vi "Eye Movement Analyser.vi"(7 "Data Output":T12) -> ()   [LabVIEW 2016] (continued)
          tunnel: w2511 -> [w2526]
          tunnel: w2501 -> [w2523] mode=indexing
          shift-right: [w2525] -> w2509
          shift-left: w2507 -> [w2524]
          tunnel: w2492 -> [w2522]
          # "Delete impulses marked for deletion"
          n1237 = call "Delete Impulse.vi"("Impulse Direction +ve?"=w2527, "Number of Impulses"=w2522, "Impulse Plane"=w2526, "Impulse Positions (in)"=w2524, "Plot Number"=w2523) -> ("Impulse Positions (out)"=w2525:T11)  [unwired: 14 in]
        }
        n1238 = call "Add History.vi"("Data IN"=w2506, "Impulse Positions"=w2507) -> ("Data OUT"=w2505:T30)  [unwired: 9 in]
        n1239 = disable-structure shown="Enabled" {
          disable-tunnel: w2492 -> [w2517 w2521]
          disable-tunnel: w2501 -> [w2516 _]
          disable-tunnel: [w2514 w2521] -> w2500
          frame Disabled {
            # "Calc new No. Imp"
            # "Keep selected trace value less than number of impulses."
            n1240 = Array Size(array=w2516) -> (size(s)=w2515:i32)
            n1241 = Subtract(x=w2517, y=w2515) -> (x-y=w2514:i32)
            n1242 = local read "Trace"() -> (w2520:i32)
            n1243 = Decrement(x=w2514) -> (x-1=w2518:i32)
            n1244 = Max & Min(x=w2520, y=w2518) -> (min(x,y)=w2519:i32)  [unwired: 1 out]
            n1245 = local write "Trace"(w2519) -> ()
          }
          frame Enabled {
          }
        }
        n1246 = local write "Impulse Positions"(w2509) -> ()
        n1247 = Bundle By Name(cluster=w2505, "Impulse Positions"=w2509, "No. Imp"=w2500) -> (w2510:T30)
      }
      frame "Cut Before" {
        n1248 = local read "Impulse Plane 2"() -> (w2540:T9)
        n1249 = local read "Impulse dir"() -> (w2541:bool)
        n1250 = Unbundle By Name(w2530) -> ("Impulse Positions"=w2531:T11)
        n1251 = property on="Impulse Trace" class="WFGraph (strict)"() -> ("Cursor.Cursor Position:Cursor X"=w2537:dbl)  [unwired: 2 in, 2 out]
        n1252 = local read "Data Output"() -> (w2534:T12)
        n1253 = Unbundle By Name(w2534) -> ("Sample Rate"=w2535:i32)
        n1254 = call "Cut Impulse.vi"("Sample Rate"=w2535, "Impulse Direction +ve?"=w2541, "Cut region"=enum16{"Before", "After"}."Before", "X Position"=w2537, "Impulse Plane"=w2540, "Impulse Positions (in)"=w2531) -> ("Impulse Positions (out)"=w2538:T11)  [unwired: 13 in]
        n1255 = local write "Impulse Positions"(w2538) -> ()
        n1256 = call "Add History.vi"("Data IN"=w2530, "Impulse Positions"=w2531) -> ("Data OUT"=w2529:T30)  [unwired: 9 in]
        n1257 = Bundle By Name(cluster=w2529, "Impulse Positions"=w2538) -> (w2539:T30)
      }
      frame "Cut After" {
        n1258 = local read "Impulse Plane 2"() -> (w2555:T9)
        n1259 = local read "Data Output"() -> (w2549:T12)
        n1260 = local read "Impulse dir"() -> (w2556:bool)
        n1261 = Unbundle By Name(w2545) -> ("Impulse Positions"=w2546:T11)
        n1262 = property on="Impulse Trace" class="WFGraph (strict)"() -> ("Cursor.Cursor Position:Cursor X"=w2552:dbl)  [unwired: 2 in, 2 out]
        n1263 = Unbundle By Name(w2549) -> ("Sample Rate"=w2550:i32)
        n1264 = call "Cut Impulse.vi"("Sample Rate"=w2550, "Impulse Direction +ve?"=w2556, "Cut region"=enum16{"Before", "After"}."After", "X Position"=w2552, "Impulse Plane"=w2555, "Impulse Positions (in)"=w2546) -> ("Impulse Positions (out)"=w2553:T11)  [unwired: 13 in]
        n1265 = local write "Impulse Positions"(w2553) -> ()
        n1266 = call "Add History.vi"("Data IN"=w2545, "Impulse Positions"=w2546) -> ("Data OUT"=w2544:T30)  [unwired: 9 in]
        n1267 = Bundle By Name(cluster=w2544, "Impulse Positions"=w2553) -> (w2554:T30)
      }
      frame "Cut in Range" {
        n1268 = stacked-sequence {
          tunnel: [_ w2578 _ _] -> w2563
          tunnel: [_ _ _ w2580] -> w2564
          frame #0 {
            n1269 = property on="Time series Trace" class="WFGraph (strict)"("Active Cursor"=u32 0) -> ()  [unwired: 2 in, 2 out]
          }
          frame #1 {
            n1270 = property on="Time series Trace" class="WFGraph (strict)"() -> ("Cursor.Cursor Position:Cursor X"=w2578:dbl)  [unwired: 2 in, 2 out]
          }
          frame #2 {
            n1271 = property on="Time series Trace" class="WFGraph (strict)"("Active Cursor"=u32 1) -> ()  [unwired: 2 in, 2 out]
          }
          frame #3 {
            n1272 = property on="Time series Trace" class="WFGraph (strict)"() -> ("Cursor.Cursor Position:Cursor X"=w2580:dbl)  [unwired: 2 in, 2 out]
          }
        }
        n1273 = Unbundle By Name(w2561) -> ("Data File.Data Channels"=w2572:dbl[][], "Data File.Sample Rate"=w2567:i32)
        n1274 = Less?(x=w2563, y=w2564) -> (x < y?=w2566:bool)
        n1275 = case shown="True" w2566 {
          tunnel: w2564 -> [_ w2592]
          tunnel: w2572 -> [_ w2589]
          tunnel: [dbl[][] [] w2583] -> w2569
          tunnel: w2567 -> [_ w2582]
          frame False {
          }
          frame True {
            n1276 = Multiply(x=w2582, y=w2592) -> (x*y=w2591:dbl)
            n1277 = To Long Integer(number=w2591) -> (32bit integer=w2584:i32)
            n1278 = Array Size(array=w2589) -> (size(s)=w2588:i32[])
            n1279 = Index Array(array=w2588, index=1) -> (element=w2586:i32)
            n1280 = Subtract(x=w2586, y=w2584) -> (x-y=w2585:i32)
            n1281 = Array Subset(array=w2589, index (col)=w2584, length (col)=w2585) -> (w2590:dbl[][])  [unwired: 2 in]
            n1282 = Transpose 2D Array(2D array=w2590) -> (transposed array=w2583:dbl[][])
          }
        }
        n1283 = Multiply(x=w2567, y=w2563) -> (x*y=w2575:dbl)
        n1284 = To Long Integer(number=w2575) -> (32bit integer=w2570:i32)
        n1285 = Array Subset(array=w2572, index (col)=0 ("index"), length (col)=w2570) -> (w2574:dbl[][])  [unwired: 2 in]
        n1286 = Transpose 2D Array(2D array=w2574) -> (transposed array=w2568:dbl[][])
        n1287 = Build Array (concatenate)(w2568, w2569) -> (w2573:dbl[][])
        n1288 = Transpose 2D Array(2D array=w2573) -> (transposed array=w2565:dbl[][])
        n1289 = Bundle By Name(cluster=w2561, "Data File.Data Channels"=w2565) -> (w2560:T30)
      }
      frame "Keep in range" {
        n1290 = flat-sequence {
          tunnel: [w2611] -> w2605
          tunnel: [w2609] -> w2600
          tunnel: [w2608] -> w2599
          tunnel: w2597 -> [w2607]
          tunnel: w2605 -> [w2626]
          tunnel: [w2626] -> w2604
          tunnel: [T12 {"Data Channels"=[], "Sample Rate"=0, "Channel List"=[]} ("Data Output")] -> w2603
          tunnel: [w2624] -> w2602
          tunnel: w2599 -> [w2624]
          tunnel: [w2623] -> w2601
          tunnel: w2600 -> [w2623]
          tunnel: w2604 -> [w2628]
          tunnel: w2603 -> [w2631]
          tunnel: w2602 -> [w2630]
          tunnel: w2601 -> [w2629]
          tunnel: [w2627] -> w2595
          frame #0 {
            n1291 = Unbundle By Name(w2607) -> ("Data File.Channel List"=w2609:string[], "Data File.Data Channels"=w2613:dbl[][], "Data File.Sample Rate"=w2608:i32)
            n1292 = stacked-sequence {
              tunnel: [_ w2620 _ _] -> w2616
              tunnel: [_ _ _ w2622] -> w2615
              frame #0 {
                n1293 = property on="Time series Trace" class="WFGraph (strict)"("Active Cursor"=u32 0) -> ()  [unwired: 2 in, 2 out]
              }
              frame #1 {
                n1294 = property on="Time series Trace" class="WFGraph (strict)"() -> ("Cursor.Cursor Position:Cursor X"=w2620:dbl)  [unwired: 2 in, 2 out]
              }
              frame #2 {
                n1295 = property on="Time series Trace" class="WFGraph (strict)"("Active Cursor"=u32 1) -> ()  [unwired: 2 in, 2 out]
              }
              frame #3 {
                n1296 = property on="Time series Trace" class="WFGraph (strict)"() -> ("Cursor.Cursor Position:Cursor X"=w2622:dbl)  [unwired: 2 in, 2 out]
              }
            }
            n1297 = Subtract(x=w2615, y=w2616) -> (x-y=w2617:dbl)
            n1298 = Multiply(x=w2608, y=w2616) -> (x*y=w2612:dbl)
            n1299 = Multiply(x=w2608, y=w2617) -> (x*y=w2618:dbl)
            n1300 = To Long Integer(number=w2612) -> (32bit integer=w2614:i32)
            n1301 = To Long Integer(number=w2618) -> (32bit integer=w2610:i32)
            n1302 = Array Subset(array=w2613, index (col)=w2614, length (col)=w2610) -> (w2611:dbl[][])  [unwired: 2 in]
          }
          frame #1 {
          }
          frame #2 {
            n1303 = Bundle By Name(cluster=w2631, "Channel List"=w2629, "Data Channels"=w2628, "Sample Rate"=w2630) -> (w2627:T12)
          }
        }
        n1304 = Bundle By Name(cluster=w2597, "Data File"=w2595) -> (w2596:T30)
      }
      frame "Undo Last" {
        n1305 = Unbundle By Name(w2637) -> ("Undo Counter"=w2636:i32, "Impulse Positions"=w2638:T11)
        n1306 = case shown="0" w2636 {
          tunnel: w2638 -> [w2651 _]
          tunnel: w2637 -> [w2650 w2652]
          tunnel: [w2648 w2652] -> w2633
          frame 0 {
            n1307 = call "Add History.vi"("Data IN"=w2650, "Impulse Positions"=w2651) -> ("Data OUT"=w2649:T30)  [unwired: 9 in]
            n1308 = Bundle By Name(cluster=w2649, "Undo Counter"=1) -> (w2648:T30)
          }
          frame 1.., Default {
          }
        }
        n1309 = Unbundle By Name(w2633) -> ("Old Impulse positions for Undo"=w2644:T35, "Undo Counter"=w2635:i32, "History Length"=w2642:i32, "Histpry Position"=w2643:i32)
        n1310 = Increment(x=w2635) -> (x+1=w2639:i32)
        n1311 = Less?(x=w2639, y=w2642) -> (x < y?=w2641:bool)
        n1312 = case shown="True" w2641 {
          tunnel: w2635 -> [_ w2656]
          tunnel: w2643 -> [_ w2665]
          tunnel: w2642 -> [_ w2662]
          tunnel: w2644 -> [_ w2661]
          tunnel: w2633 -> [w2653 w2655]
          tunnel: [w2653 w2660] -> w2645
          frame False {
            n1313 = One Button Dialog(message="End of History") -> ()  [unwired: 1 in, 1 out]
          }
          frame True {
            n1314 = Subtract(x=w2665, y=w2656) -> (x-y=w2663:i32)
            n1315 = Less Than 0?(x=w2663) -> (x < 0?=w2664:bool)
            n1316 = case shown="False" w2664 {
              tunnel: w2663 -> [w2666 w2669]
              tunnel: w2662 -> [_ w2668]
              tunnel: [w2666 w2667] -> w2657
              frame False {
              }
              frame True {
                n1317 = Add(x=w2669, y=w2668) -> (x+y=w2667:i32)
              }
            }
            n1318 = Index Array(array=w2661, index (row)=w2657) -> (element=w2659:T11)  [unwired: 1 in]
            n1319 = Increment(x=w2656) -> (x+1=w2658:i32)
            n1320 = local write "Impulse Positions"(w2659) -> ()
            n1321 = Bundle By Name(cluster=w2655, "Impulse Positions"=w2659, "Undo Counter"=w2658) -> (w2660:T30)
          }
        }
      }
      frame "Redo" {
        n1322 = Unbundle By Name(w2677) -> ("Old Impulse positions for Undo"=w2676:T35, "Undo Counter"=w2672:i32, "History Length"=w2674:i32, "Histpry Position"=w2675:i32)
        n1323 = Decrement(x=w2672) -> (x-1=w2671:i32)
        n1324 = Greater Than 0?(x=w2671) -> (x > 0?=w2673:bool)
        n1325 = case shown="True" w2673 {
          tunnel: w2671 -> [_ w2686]
          tunnel: w2675 -> [_ w2694]
          tunnel: w2674 -> [_ w2691]
          tunnel: w2676 -> [_ w2690]
          tunnel: w2677 -> [w2682 w2689]
          tunnel: [w2682 w2688] -> w2680
          frame False {
            n1326 = One Button Dialog(message="Current Data") -> ()  [unwired: 1 in, 1 out]
          }
          frame True {
            n1327 = Subtract(x=w2694, y=w2686) -> (x-y=w2692:i32)
            n1328 = Less Than 0?(x=w2692) -> (x < 0?=w2693:bool)
            n1329 = case shown="True" w2693 {
              tunnel: w2692 -> [w2695 w2698]
              tunnel: w2691 -> [_ w2697]
              tunnel: [w2695 w2696] -> w2685
              frame False {
              }
              frame True {
                n1330 = Add(x=w2698, y=w2697) -> (x+y=w2696:i32)
              }
            }
            n1331 = Increment(x=w2685) -> (x+1=w2684:i32)
            n1332 = Index Array(array=w2690, index (row)=w2684) -> (element=w2687:T11)  [unwired: 1 in]
            n1333 = local write "Impulse Positions"(w2687) -> ()
            n1334 = Bundle By Name(cluster=w2689, "Impulse Positions"=w2687, "Undo Counter"=w2686) -> (w2688:T30)
          }
        }
      }
      frame "Filter Data" {
        n1335 = Unbundle By Name(w2700) -> ("Data File"=w2701:T12)
        n1336 = Unbundle By Name(w2701) -> ("Data Channels"=w2705:dbl[][], "Sample Rate"=w2711:i32)
        n1337 = local read "Interpolate"() -> (w2704:bool)
        n1338 = Unbundle By Name("Filter characteristics") -> ("Lower pass freq"=w2708:dbl, "Higher pass freq"=w2709:dbl, "Filter type"=w2712:T52, "Order"=w2710:i32)
        n1339 = case shown="True" w2704 {
          tunnel: w2705 -> [w2715 w2718]
          tunnel: [w2715 w2717] -> w2706
          frame False {
            # "Do nothing."
          }
          frame True {
            # "Interpolate without\nremoving front and end data."
            n1340 = call "interp type 2.vi"("NaN"=w2718, "Remove front and end"=FALSE) -> ("Interpolated"=w2717:dbl[][])
          }
        }
        n1341 = call "FIR filter neu.vi"("order"=w2710, "filter type"=w2712, "higher pass freq"=w2709, "lower pass freq"=w2708, "sampling freq: fs"=w2711, "3D Unfiltered Data"=w2706) -> ("Output Array"=w2707:dbl[][])  [unwired: 3 in]
        n1342 = Bundle By Name(cluster=w2700, "Data File.Data Channels"=w2707) -> (w2699:T30)
      }
      frame "Generate New Time Plot" {
        n1343 = Unbundle By Name(w2720) -> ("Data File.Sample Rate"=w2726:i32, "Parameter Time Series"=w2724:T2)
        n1344 = for {
          tunnel: w2724 -> [w2826] mode=indexing
          tunnel: w2720 -> [w2823]
          shift-right: [w2825] -> w2729
          shift-left: dbl[][] [] -> [w2824]
          tunnel: w2726 -> [w2811]
          n1345 = Unbundle By Name(w2826) -> ("List 1"=w2821:u16, "inverse"=w2820:bool, "Gain"=w2815:dbl, "Offset"=w2816:dbl, "time offset"=w2813:dbl, "interpolate"=w2808:bool)
          n1346 = Unbundle By Name(w2823) -> ("Data File.Data Channels"=w2822:dbl[][])
          n1347 = Index Array(array=w2822, index (row)=w2821) -> (element=w2817:dbl[])  [unwired: 1 in]
          n1348 = Multiply(x=w2817, y=w2815) -> (x*y=w2818:dbl[])
          n1349 = case shown="False" w2820 {
            tunnel: w2818 -> [w2830 w2832]
            tunnel: [w2830 w2831] -> w2819
            frame False {
            }
            frame True {
              n1350 = Negate(x=w2832) -> (-x=w2831:dbl[])
            }
          }
          n1351 = Add(x=w2819, y=w2816) -> (x+y=w2814:dbl[])
          n1352 = Multiply(x=w2811, y=w2813) -> (x*y=w2812:dbl)
          n1353 = Split 1D Array(array=w2814, index=w2812) -> (second subarray=w2810:dbl[])  [unwired: 1 out]
          n1354 = case shown="False" w2808 {
            tunnel: w2810 -> [w2827 w2829]
            tunnel: [w2827 w2828] -> w2809
            frame False {
            }
            frame True {
              n1355 = call "interp type 2 1D.vi"("NaN"=w2829) -> ("Interpolated"=w2828:dbl[])
            }
          }
          n1356 = Build Array (concatenate)(w2824, w2809) -> (w2825:dbl[][])
        }
        n1357 = case shown="True" "Interpolate" {
          tunnel: w2729 -> [w2732 w2735]
          tunnel: [w2732 w2734] -> w2728
          frame False {
          }
          frame True {
            n1358 = call "interp type 2.vi"("NaN"=w2735, "Remove front and end"=TRUE) -> ("Interpolated"=w2734:dbl[][])
          }
        }
        n1359 = stacked-sequence {
          tunnel: w2728 -> [_ _ w2748 _]
          tunnel: w2724 -> [_ _ _ w2792]
          tunnel: w2726 -> [_ _ w2747 _]
          tunnel: w2720 -> [_ _ w2744 _]
          frame #0 {
            n1360 = case shown="False" "Fixed Amplitude 2" {
              tunnel: [u8 0 ("Y Scale.Scale Fit") u8 2 ("Y Scale.Scale Fit")] -> w2736
              frame True {
              }
              frame False {
              }
            }
            n1361 = property on="Time series Trace" class="WFGraph (strict)"("Y Scale.Scale Fit"=w2736) -> ()  [unwired: 2 in, 2 out]
          }
          frame #1 {
            n1362 = case shown="False" "Fixed Time 2" {
              tunnel: [u8 0 ("Y Scale.Scale Fit") u8 2 ("Y Scale.Scale Fit")] -> w2741
              frame True {
              }
              frame False {
              }
            }
            n1363 = property on="Time series Trace" class="WFGraph (strict)"("X Scale.Scale Fit"=w2741) -> ()  [unwired: 2 in, 2 out]
          }
          frame #2 {
            n1364 = Reciprocal(x=w2747) -> (1/x=w2749:dbl)
            n1365 = case shown="True" "Gl Spline" {
              tunnel: w2748 -> [w2756 w2765]
              tunnel: [w2755 w2766] -> w2745
              tunnel: w2747 -> [_ w2767]
              tunnel: w2744 -> [w2754 _]
              frame False {
                n1366 = Unbundle By Name(w2754) -> ("desacc"=w2753:T31, "Data File.Sample Rate"=w2752:i32)
                n1367 = disable-structure shown="Enabled" {
                  disable-tunnel: w2756 -> [w2762 w2763]
                  disable-tunnel: [w2761 w2763] -> w2755
                  disable-tunnel: w2753 -> [w2759 _]
                  disable-tunnel: w2752 -> [w2758 _]
                  frame Disabled {
                    n1368 = call "desacade.vi"("Data not diff"=w2762, "Capture Saccades"=FALSE, "desacc"=w2759, "Sample Rate"=w2758, "Display Saccades"=FALSE) -> ("Desaccaded"=w2761:dbl[][])  [unwired: 5 in, 5 out]
                  }
                  frame Enabled {
                  }
                }
              }
              frame True {
                n1369 = local read "Interpolate"() -> (w2768:bool)
                n1370 = case shown="False" w2768 {
                  tunnel: w2765 -> [w2790 w2791]
                  tunnel: [w2789 w2791] -> w2764
                  frame False {
                    n1371 = call "interp type 2.vi"("NaN"=w2790, "Remove front and end"=TRUE) -> ("Interpolated"=w2789:dbl[][])
                  }
                  frame True {
                  }
                }
                n1372 = for {
                  tunnel: w2767 -> [w2783]
                  tunnel: w2764 -> [w2770] mode=indexing
                  tunnel: [w2772] -> w2766 mode=indexing
                  n1373 = Array Size(array=w2770) -> (size(s)=w2786:i32)
                  n1374 = Decrement(x=w2786) -> (x-1=w2785:i32)
                  n1375 = call-poly <vilib>:"Ramp Pattern.vi"("start"=0.0, "end"=w2785, "samples"=w2786) -> ("Ramp Pattern"=w2784:dbl[])  [unwired: 7 in, 1 out]
                  n1376 = Divide(x=w2784, y=w2783) -> (x/y=w2780:dbl[])
                  n1377 = call-poly <vilib>:"Mean.vi"("X"=w2770) -> ("mean"=w2771:dbl)  [unwired: 1 out]
                  n1378 = call <vilib>:"Cubic Spline Fit.vi"("Y"=w2770, "X"=w2780, "balance parameter"="Spline balance parameter") -> ("Best Cubic Spline Fit"=w2772:dbl[])  [unwired: 11 in, 1 out]
                  n1379 = Subtract(x=w2772, y=w2770) -> (x-y=w2781:dbl[])
                  n1380 = Subtract(x=w2770, y=w2771) -> (x-y=w2778:dbl[])
                  n1381 = Multiply(x=w2781, y=w2781) -> (x*y=w2782:dbl[])
                  n1382 = Multiply(x=w2778, y=w2778) -> (x*y=w2779:dbl[])
                  n1383 = Add Array Elements(numeric array=w2782) -> (sum=w2777:dbl)
                  n1384 = Add Array Elements(numeric array=w2779) -> (sum=w2776:dbl)
                  n1385 = Divide(x=w2777, y=w2776) -> (x/y=w2775:dbl)
                  n1386 = Negate(x=w2775) -> (-x=w2774:dbl)
                  n1387 = Increment(x=w2774) -> (x+1=→"R-sq":dbl)
                }
              }
            }
            n1388 = Bundle(0.0, w2749, "Best Cubic Spline Fit"=w2745) -> (→"Time series Trace":T53)  [unwired: 1 in]
          }
          frame #3 {
            n1389 = for {
              tunnel: w2792 -> [w2796] mode=indexing
              i -> [w2795]
              n1390 = Unbundle By Name(w2796) -> ("Color Box"=w2794:u32, "Boolean"=w2793:bool)
              n1391 = stacked-sequence {
                tunnel: w2795 -> [w2797 _]
                tunnel: w2793 -> [_ w2803]
                tunnel: w2794 -> [_ w2802]
                frame #0 {
                  n1392 = property on="Time series Trace" class="WFGraph (strict)"("Active Plot"=w2797) -> ()  [unwired: 2 in, 2 out]
                }
                frame #1 {
                  n1393 = local read "Interpolate"() -> (w2799:bool)
                  n1394 = case shown="False" w2799 {
                    tunnel: [u8 2 ("Plot.Point Style") u8 4 ("Plot.Point Style")] -> w2798
                    frame False {
                    }
                    frame True {
                    }
                  }
                  n1395 = case shown="False" "Dots" {
                    tunnel: [u8 0 ("Plot.Point Style") u8 2 ("Plot.Point Style")] -> w2801
                    frame False {
                    }
                    frame True {
                    }
                  }
                  n1396 = property on="Time series Trace" class="WFGraph (strict)"("Plot.Plot Color"=w2802, "Plot.Visible"=w2803, "Plot.Plot Interpolation"=w2798, "Plot.Point Style"=w2801, "Plot.Fill/Pt. Color"=w2802) -> ()  [unwired: 2 in, 2 out]
                }
              }
            }
          }
        }
        n1397 = Bundle By Name(cluster=w2723, "Session saved?"=FALSE) -> (w2722:T17)
      }
      frame "Make off and gains permanent" {
        n1398 = local read "Parameter Time Series"() -> (w2854:T2)
        n1399 = local read "Data Output"() -> (w2853:T12)
        n1400 = Unbundle By Name(w2853) -> ("Sample Rate"=w2855:i32)
        n1401 = for {
          tunnel: w2854 -> [w2873] mode=indexing
          tunnel: w2855 -> [w2863]
          shift-right: [w2857] -> w2837
          shift-left: w2853 -> [w2862]
          n1402 = Unbundle By Name(w2873) -> ("List 1"=w2860:u16, "inverse"=w2872:bool, "Gain"=w2867:dbl, "Offset"=w2868:dbl, "time offset"=w2865:dbl)
          n1403 = Unbundle By Name(w2862) -> ("Data Channels"=w2861:dbl[][])
          n1404 = Index Array(array=w2861, index (row)=w2860) -> (element=w2869:dbl[])  [unwired: 1 in]
          n1405 = Multiply(x=w2869, y=w2867) -> (x*y=w2870:dbl[])
          n1406 = case shown="True" w2872 {
            tunnel: w2870 -> [w2874 w2876]
            tunnel: [w2874 w2875] -> w2871
            frame False {
            }
            frame True {
              n1407 = Negate(x=w2876) -> (-x=w2875:dbl[])
            }
          }
          n1408 = Add(x=w2871, y=w2868) -> (x+y=w2866:dbl[])
          n1409 = Multiply(x=w2863, y=w2865) -> (x*y=w2864:dbl)
          n1410 = Split 1D Array(array=w2866, index=w2864) -> (second subarray=w2859:dbl[])  [unwired: 1 out]
          n1411 = Replace Array Subset(array=w2861, new element=w2859, index (row)=w2860) -> (w2858:dbl[][])  [unwired: 1 in]
          n1412 = Bundle By Name(cluster=w2862, "Data Channels"=w2858) -> (w2857:T12)
        }
        n1413 = File Dialog(7:"Please Enter Name Of File (NO Postfix):" ("prompt")) -> (0:w2839:errorcluster, 3:w2844:path)  [unwired: 6 in, 2 out]
        n1414 = Unbundle(w2839) -> ()  [unwired: 3 out]
        n1415 = Bundle("Data Output"=w2837, "Data OUT"=w2836) -> (w2838:T39)  [unwired: 1 in]
        n1416 = Path To String(path=w2844) -> (string=w2842:string)
        n1417 = call "File-Suffix.vi"("Substring"=".lvs-e", "String 2"=w2842) -> ("String"=w2840:string)
        n1418 = String To Path(string=w2840) -> (path=w2850:path)
        n1419 = Flatten To String(anything=w2838) -> (data string=w2847:string)  [unwired: 3 in, 2 out]
        n1420 = call <vilib>:"Open_Create_Replace File.vi"("function (open:0)"=T19."create or replace", "file path"=w2850) -> ("refnum"=w2845:refnum<file>)  [unwired: 6 in, 3 out]
        n1421 = String Length(string=w2847) -> (length=w2849:i32)
        n1422 = Flatten To String(anything=w2849) -> (data string=w2848:string)  [unwired: 3 in, 2 out]
        n1423 = call <vilib>:"Write File+ (string).vi"("string"=w2848, "refnum"=w2845) -> ("dup refnum"=w2846:refnum<file>)  [unwired: 5 in, 2 out]
        n1424 = call <vilib>:"Write File+ (string).vi"("string"=w2847, "refnum"=w2846) -> ("dup refnum"=w2852:refnum<file>)  [unwired: 5 in, 2 out]
        n1425 = call <vilib>:"Close File+.vi"("refnum"=w2852) -> ()  [unwired: 4 in, 3 out]
      }
      frame "Export Data" {
        n1426 = stacked-sequence {
          seq-local: [w2899 _] -> [_ w2966]
          seq-local: [w2895 _] -> [_ w2959]
          tunnel: w2880 -> [w2905 _]
          frame #0 {
            w2893 = TRUE ("Mean and STD")
            (unwired) T54."new or existing file" ("select mode (2)")
            w2906 = "\r"
            w2922 = "\r"
            n1427 = local read "Parameter Impuls Series"() -> (w2930:T8)
            n1428 = local read "Data Output"() -> (w2884:T12)
            n1429 = Unbundle By Name(w2905) -> ("Impulse Positions"=w2933:T11, "desacc"=w2882:T31)
            n1430 = Unbundle By Name(w2884) -> ("Sample Rate"=w2885:i32, "Channel List"=w2883:string[])
            n1431 = Index Array(array=w2930, index=0 ("Index")) -> (element=w2928:T55)
            n1432 = Array Size(array=w2883) -> (size(s)=w2918:i32)
            n1433 = for {
              tunnel: w2928 -> [w2946]
              tunnel: [w2945] -> w2927 mode=indexing
              shift-right: [w2943] -> w2907
              shift-left: "" -> [w2944]
              tunnel: w2883 -> [w2942] mode=indexing
              i -> [w2938]
              n1434 = local read "Parameter Impuls Series"() -> (w2939:T8)
              n1435 = for {
                tunnel: w2939 -> [w2953] mode=indexing
                tunnel: w2938 -> [w2951]
                shift-right: [w2948] -> w2936
                shift-left: FALSE ("Boolean 3") -> [w2949]
                n1436 = Unbundle By Name(w2953) -> ("Channel"=w2952:u16, "Desaccade"=w2947:bool)
                n1437 = Equal?(x=w2951, y=w2952) -> (x = y?=w2950:bool)
                n1438 = case shown="True" w2950 {
                  tunnel: w2949 -> [w2954 _]
                  tunnel: [w2954 w2955] -> w2948
                  tunnel: w2947 -> [_ w2955]
                  frame False {
                  }
                  frame True {
                  }
                }
              }
              n1439 = Bundle By Name(cluster=w2946, "Gain"=1.0, "Offset"=0.0, "Invert"=FALSE ("Boolean 2"), "Channel"=w2938, "Desaccade"=w2936) -> (w2945:T55)
              n1440 = Concatenate Strings(w2944, w2942, "\t") -> (w2943:string)
            }
            n1441 = Format Into String(format string="%d" ("Format String"), w2918) -> (resulting string=w2916:string)  [unwired: 2 in, 1 out]
            n1442 = local read "Impulse Plane 2"() -> (w2931:T9)
            n1443 = local read "Impulse dir"() -> (w2932:bool)
            n1444 = To Double Precision Float(number=w2885) -> (double precision float=w2926:dbl)
            n1445 = local read "Interpolate"() -> (w2889:bool)
            n1446 = Unbundle By Name(w2884) -> ("Sample Rate"=w2896:i32, "Channel List"=w2897:string[])
            n1447 = Format Into String(format string="%d" ("Format String"), w2926) -> (resulting string=w2924:string)  [unwired: 2 in, 1 out]
            n1448 = local read "S-pline"() -> (w2886:bool)
            n1449 = Concatenate Strings("Number of Channels " ("Substring"), w2916, w2906, "Channel  Names " ("Substring"), w2906, w2907) -> (w2923:string)
            n1450 = Concatenate Strings("Sample Rate ", w2924, w2922, w2923, w2922) -> (w2909:string)
            n1451 = local read "Spline balance parameter"() -> (w2887:dbl)
            n1452 = call "Couple Head Impulse Traces.vi"("Data Input"=w2884, "Impulse Positions"=w2933, "Impulse Direction +ve?"=w2932, "Impulse Plane"=w2931, "Mean and STD"=w2893, "Plot Selection 2"=w2927, "Export"=w2893, "desacc"=w2882, "Interpolate"=w2889, "S-pline"=w2886, "balance parameter (s-pline Parameter)"=w2887) -> ("Mean and STD"=w2894:dbl[][])  [unwired: 5 in, 3 out]
            n1453 = File Dialog(7:"Please Enter Name Of File (NO Postfix):" ("prompt")) -> (0:w2888:errorcluster, 3:w2899:path)  [unwired: 6 in, 2 out]
            n1454 = Transpose 2D Array "Means"(2D array=w2894) -> (transposed array=w2915:dbl[][])
            n1455 = local read "Data Output"() -> (w2898:T12)
            n1456 = Bundle By Name(cluster=w2898, "Data Channels"=w2894, "Sample Rate"=w2896, "Channel List"=w2897) -> (w2895:T12)
            n1457 = Unbundle(w2888) -> ()  [unwired: 3 out]
            n1458 = Path To String(path=w2899) -> (string=w2891:string)
            n1459 = call "File-Suffix.vi"("Substring"=".txt", "String 2"=w2891) -> ("String"=w2890:string)
            n1460 = Array To Spreadsheet String(delimiter (Tab)="\t", array=w2915, 3:"%.5f" ("format string")) -> (spreadsheet string=w2912:string)
            n1461 = String To Path(string=w2890) -> (path=w2900:path)
            n1462 = call <vilib>:"Open_Create_Replace File.vi"("function (open:0)"=T19."create or replace", "file path"=w2900) -> ("error out"=w2904:errorcluster, "refnum"=w2903:refnum<file>)  [unwired: 6 in, 2 out]
            n1463 = call <vilib>:"Write File+ (string).vi"("string"=w2909, "error in (no error)"=w2904, "refnum"=w2903) -> ("dup refnum"=w2911:refnum<file>)  [unwired: 4 in, 2 out]
            n1464 = call <vilib>:"Write File+ (string).vi"("string"=w2912, "refnum"=w2911) -> ("dup refnum"=w2910:refnum<file>)  [unwired: 5 in, 2 out]
            n1465 = call <vilib>:"Close File+.vi"("refnum"=w2910) -> ()  [unwired: 4 in, 3 out]
          }
          frame #1 {
            n1466 = Path To String(path=w2966) -> (string=w2957:string)
            n1467 = call "File-Suffix.vi"("Substring"=".lvd", "String 2"=w2957) -> ("String"=w2958:string)
            n1468 = String To Path(string=w2958) -> (path=w2965:path)
            n1469 = Flatten To String(anything=w2959) -> (data string=w2962:string)  [unwired: 3 in, 2 out]
            n1470 = call <vilib>:"Open_Create_Replace File.vi"("function (open:0)"=T19."create or replace", "file path"=w2965) -> ("refnum"=w2960:refnum<file>)  [unwired: 6 in, 3 out]
            n1471 = String Length(string=w2962) -> (length=w2964:i32)
            n1472 = Flatten To String(anything=w2964) -> (data string=w2963:string)  [unwired: 3 in, 2 out]
            n1473 = call <vilib>:"Write File+ (string).vi"("string"=w2963, "refnum"=w2960) -> ("dup refnum"=w2961:refnum<file>)  [unwired: 5 in, 2 out]
            n1474 = call <vilib>:"Write File+ (string).vi"("string"=w2962, "refnum"=w2961) -> ("dup refnum"=w2968:refnum<file>)  [unwired: 5 in, 2 out]
            n1475 = call <vilib>:"Close File+.vi"("refnum"=w2968) -> ()  [unwired: 4 in, 3 out]
          }
        }
      }
      frame "Export Time Series Data" {
        (unwired) T54."new or existing file" ("select mode (2)")
        w2983 = "\r"
        (unwired) T54."new or existing file" ("select mode (2)")
        n1476 = local read "Parameter Time Series"() -> (w2977:T2)
        n1477 = local read "Data Output"() -> (w2973:T12)
        n1478 = for {
          tunnel: w2977 -> [w3020] mode=indexing
          tunnel: w2973 -> [w3017]
          shift-right: [w3019] -> w3002
          shift-left: dbl[][] [] -> [w3018]
          shift-right: [w3014] -> w2981
          shift-left: _ -> [w3015]
          n1479 = Unbundle By Name(w3020) -> ("List 1"=w3012:u16)
          n1480 = Unbundle By Name(w3017) -> ("Channel List"=w3013:string[], "Data Channels"=w3016:dbl[][])
          n1481 = Index Array(array=w3016, index (row)=w3012) -> (element=w3009:dbl[])  [unwired: 1 in]
          n1482 = Index Array(array=w3013, index=w3012) -> (element=w3011:string)
          n1483 = Concatenate Strings(w3015, w3011, "\t") -> (w3014:string)
          n1484 = Build Array (concatenate)(w3018, w3009) -> (w3019:dbl[][])
        }
        n1485 = Unbundle By Name(w2973) -> ("Sample Rate"=w2986:i32)
        n1486 = To Double Precision Float(number=w2986) -> (double precision float=w2985:dbl)
        n1487 = local read "Interpolate"() -> (w2976:bool)
        n1488 = Format Into String(format string="%d" ("Format String"), w2985) -> (resulting string=w2984:string)  [unwired: 2 in, 1 out]
        n1489 = case shown="True" w2976 {
          tunnel: w3002 -> [w3005 w3008]
          tunnel: [w3005 w3007] -> w2979
          frame False {
          }
          frame True {
            n1490 = call "interp type 2.vi"("NaN"=w3008, "Remove front and end"=TRUE) -> ("Interpolated"=w3007:dbl[][])
          }
        }
        n1491 = Concatenate Strings("Sample Rate ", w2984, w2983, "Channel  Names " ("Substring"), w2983, w2981, w2983) -> (w2980:string)
        n1492 = File Dialog(7:"Please Enter Name Of File (NO Postfix):" ("prompt")) -> (0:w2974:errorcluster, 3:w2992:path)  [unwired: 6 in, 2 out]
        n1493 = Unbundle(w2974) -> ()  [unwired: 3 out]
        n1494 = Transpose 2D Array(2D array=w2979) -> (transposed array=w2975:dbl[][])
        n1495 = Path To String(path=w2992) -> (string=w2990:string)
        n1496 = call "File-Suffix.vi"("Substring"=".txt", "String 2"=w2990) -> ("String"=w2989:string)
        n1497 = String To Path(string=w2989) -> (path=w2993:path)
        n1498 = Array To Spreadsheet String(delimiter (Tab)="\t", array=w2975, 3:"%.5f" ("format string")) -> (spreadsheet string=w2999:string)
        n1499 = call <vilib>:"Open_Create_Replace File.vi"("function (open:0)"=T19."create or replace", "file path"=w2993) -> ("error out"=w2996:errorcluster, "refnum"=w2995:refnum<file>)  [unwired: 6 in, 2 out]
        n1500 = call <vilib>:"Write File+ (string).vi"("string"=w2980, "error in (no error)"=w2996, "refnum"=w2995) -> ("dup refnum"=w2998:refnum<file>)  [unwired: 4 in, 2 out]
        n1501 = call <vilib>:"Write File+ (string).vi"("string"=w2999, "refnum"=w2998) -> ("dup refnum"=w2997:refnum<file>)  [unwired: 5 in, 2 out]
        n1502 = call <vilib>:"Close File+.vi"("refnum"=w2997) -> ()  [unwired: 4 in, 3 out]
      }
      frame "Paint Delete" {
        n1503 = disable-structure shown="Enabled" {
          disable-tunnel: w3027 -> [w3038 _]
          disable-tunnel: [w3031 TRUE] -> w3021
          frame Disabled {
            # "Mouse down?"
            # "Cursor tool selected?"
            n1504 = Unbundle By Name(w3038) -> ("device ID"=w3040:refnum<k1>)
            n1505 = call-poly <vilib>:"Acquire Input Data.vi"("device ID"=w3040) -> ("axis info"=→"axis info":T13, "button info"=w3039:T28)  [unwired: 15 in, 2 out]
            n1506 = property on="Impulse Trace" class="WFGraph (strict)"() -> ("ActPaletteTool"=w3034:i32)  [unwired: 2 in, 2 out]
            n1507 = Unbundle By Name(w3039) -> ("button 1"=w3035:bool, "button 3"=w3036:bool)
            n1508 = Equal To 0?(x=w3034) -> (x = 0?=w3032:bool)
            n1509 = Or(x=w3035, y=w3036) -> (x .or. y?=w3033:bool)
            n1510 = And(x=w3033, y=w3032) -> (x .and. y?=w3031:bool)
          }
          frame Enabled {
          }
        }
        n1511 = Unbundle By Name(w3024) -> ("Parameter Impuls Series"=w3023:T8, "No. Imp"=w3022:i32)
        n1512 = case shown="True" w3021 {
          tunnel: [w3043 w3045] -> w3029
          tunnel: w3028 -> [w3043 w3047]
          tunnel: w3027 -> [w3042 w3053]
          tunnel: [w3042 w3052] -> w3026
          tunnel: w3023 -> [_ w3050]
          tunnel: w3022 -> [_ w3049]
          frame False {
          }
          frame True {
            w3046 = T14[] [enum."Delete Impulse", enum."Generate New Impulse Plot"] items=["--- System ---", "Panel Monitoring", "Check Save Status", "Initialize", "Initialise GUI", "Quit", "--- Import ---", "Desaccade Time Data", "Desaccade Time Data Background", "Paint Delete", "Load Batch Log File", "Make Batch List", "Update Batch List", "Delete Batch List", "Delete Temporary LVS", "Save Temporary LVS", "Check for Batch LVS", "Process 3D Chinchilla", "Find default parameter", "Mars3D old", "Chair", "EyeSeeCam", "Open last session", "Save RAW", "Auto Impulse Parameter", "Save Image", "Wireless", "Process Coils Data", "Process JHOC Data", "Process Animal Data", "Australian Data", "ASCII", "Mars 3D", "Mars 3D Training", "Position Mean Plugin", "plot generator plugin", "Human VOG system", "Optotrak", "spline", "COR", "galvanic", "Generate New Time Plot", "Make off and gains permanent", "Generate New Impulse Plot", "Defer Impulse Plot", "Fill Impulse Plot Data", "Scale Impulse Plot", "Un-Defer Impulse Plot", "Snap Impulse Cursor", "Extract Saccades", "Impulse Analyser", "NTA", "Acceleration", "Saccade Velocity", "Horizontal Align", "Vertical Align", "Delete Impulse", "Cut Before", "Cut After", "Filter Data", "Undo Last", "Redo", "Mean and STD", "Group Analyser", "Generate Report", "Phase Plots", "Gain and Phase", "Example Plugin", "Time Constant Plugin", "Export Data", "Export Time Series Data", "Append Data", "Save Data", "Load Data", "Cut in Range", "Keep in range", "Stop"]
            # "Approximation of the cursor's bounds on the plot."
            # "ms between x samples"
            n1513 = property on="Impulse Trace" class="WFGraph (strict)"() -> ("Cursor.Cursor X"=w3055:dbl, "Cursor.Cursor Y"=w3061:dbl, "YScale.Maximum"=w3066:dbl, "YScale.Minimum"=w3065:dbl)  [unwired: 2 in, 2 out]
            n1514 = property on="Impulse Trace" class="WFGraph (strict)"() -> ("Value"=w3057:cluster{dbl, dbl, "Impulses":dbl[][]})  [unwired: 2 in, 2 out]
            n1515 = Unbundle By Name(w3057) -> ("Impulses"=w3051:dbl[][])
            n1516 = Unbundle(w3057) -> (w3054:dbl)  [unwired: 2 out]
            n1517 = Subtract(x=w3066, y=w3065) -> (x-y=w3064:dbl)
            n1518 = Divide(x=w3064, y=50.0) -> (x/y=w3062:dbl)
            n1519 = Absolute Value(x=w3062) -> (abs(x)=w3060:dbl)
            n1520 = Divide(x=w3055, y=w3054) -> (x/y=w3056:dbl)
            n1521 = Add(x=w3061, y=w3060) -> (x+y=w3059:dbl)
            n1522 = Subtract(x=w3061, y=w3060) -> (x-y=w3058:dbl)
            n1523 = for {
              tunnel: w3051 -> [w3075] mode=indexing
              tunnel: w3056 -> [w3078]
              tunnel: w3059 -> [w3077]
              tunnel: w3058 -> [w3076]
              tunnel: w3050 -> [w3072]
              tunnel: w3049 -> [w3074]
              tunnel: [w3068] -> w3044 mode=indexing if=w3067
              i -> [w3068]
              # "Is the impulse visible?"
              # "If the impulse was visible and it overlaps the cursor include it for deletion."
              # "Check each impulse for deletion criteria..."
              n1524 = Divide(x=w3068, y=w3074) -> (x/y=w3073:dbl)
              n1525 = Round Toward -Infinity(1:w3073) -> (0:w3071:dbl)
              n1526 = Index Array(array=w3072, index=w3071) -> (element=w3070:T55)
              n1527 = Unbundle By Name(w3070) -> ("Visible"=w3069:bool)
              n1528 = case shown="True" w3069 {
                tunnel: w3078 -> [_ w3084]
                tunnel: w3077 -> [_ w3082]
                tunnel: w3076 -> [_ w3081]
                tunnel: [_ w3080] -> w3067
                tunnel: w3075 -> [_ w3079]
                frame False {
                  # "Impulse is not visible. Do not delete."
                }
                frame True {
                  # "Impulse is visible. Check if it intersects the cursor."
                  n1529 = Interpolate 1D Array(1:w3084, 2:w3079) -> (0:w3083:dbl)
                  n1530 = In Range and Coerce(upper limit=w3082, x=w3083, lower limit=w3081) -> (In Range?=w3080:bool)  [unwired: 1 out]
                }
              }
            }
            n1531 = Bundle By Name(cluster=w3053, "Delete-Array"=w3044) -> (w3052:T17)
            n1532 = Empty Array?(array=w3044) -> (empty?=w3048:bool)
            n1533 = Select(t=w3047, s=w3048, f=w3046) -> (s? t:f=w3045:T14[])
          }
        }
      }
    }
  }
  n1534 = stacked-sequence {
    frame #0 {
      # "GUI Inputs"
    }
    frame #1 {
    }
    frame #2 {
    }
    frame #3 {
    }
    frame #4 {
    }
  }
  n1535 = Request Deallocation(TRUE ("flag")) -> ()
